vi "5_SPA_KEYSIGHT_rabi_measurements_(SPA_Aver_Mult_traces-Rabi).vi"() -> ()   [LabVIEW 2013]
uses:
  <vilib>/Analysis/baseanly.llb/Mean (DBL).vi
  <vilib>/Analysis/NI_AALBase.lvlib
panel:
  in  "Connection":T1={"Type"=0, "VISA"="TCPIP0::192.168.0.8::inst0::INSTR", "GPIB"="10"} {"Type" items=["VISA", "GPIB"]}
  out "x/y":dbl
  out "Normalised":dbl[][](graph)
  out "(Current)":i32=103
  in  "Program to run":u16(ring) items=["Rabi", "T2"]
  in  "?":enum32{"VNA", "SPA"}(tab)
  in  "Center Freq (Hz)":dbl=6953330000.0 caption="Center Freq (Hz):" format="%#.6p"
  in  "VNA Power dBm":dbl=-10.0 caption="VNA Power (dBm)" format="%#.3f"
  in  "Points":i32=2147483647 caption="Center Freq (Hz):"
  in  "Span (Hz)":dbl=6953330000.0 caption="Center Freq (Hz):" format="%#.6p"
  in  "RBW (Hz)":dbl=6953330000.0 caption="Center Freq (Hz):" format="%#.6p"
  in  "VBW (Hz)":dbl=6953330000.0 caption="Center Freq (Hz):" format="%#.6p"
  in  "Averages":u32=251
  out "Background":dbl[][](graph)
  out "Signal":dbl[][](graph)
  out "(Current)":i32=103
  out "Background":dbl[](graph)
  in  "Numeric":u32=251
  in  "Start (ns)":dbl=2.0
  in  "End (ns)":dbl=52.0
  out "Normalised Signal":dbl[][](graph)
  out "Signal":dbl[](graph)
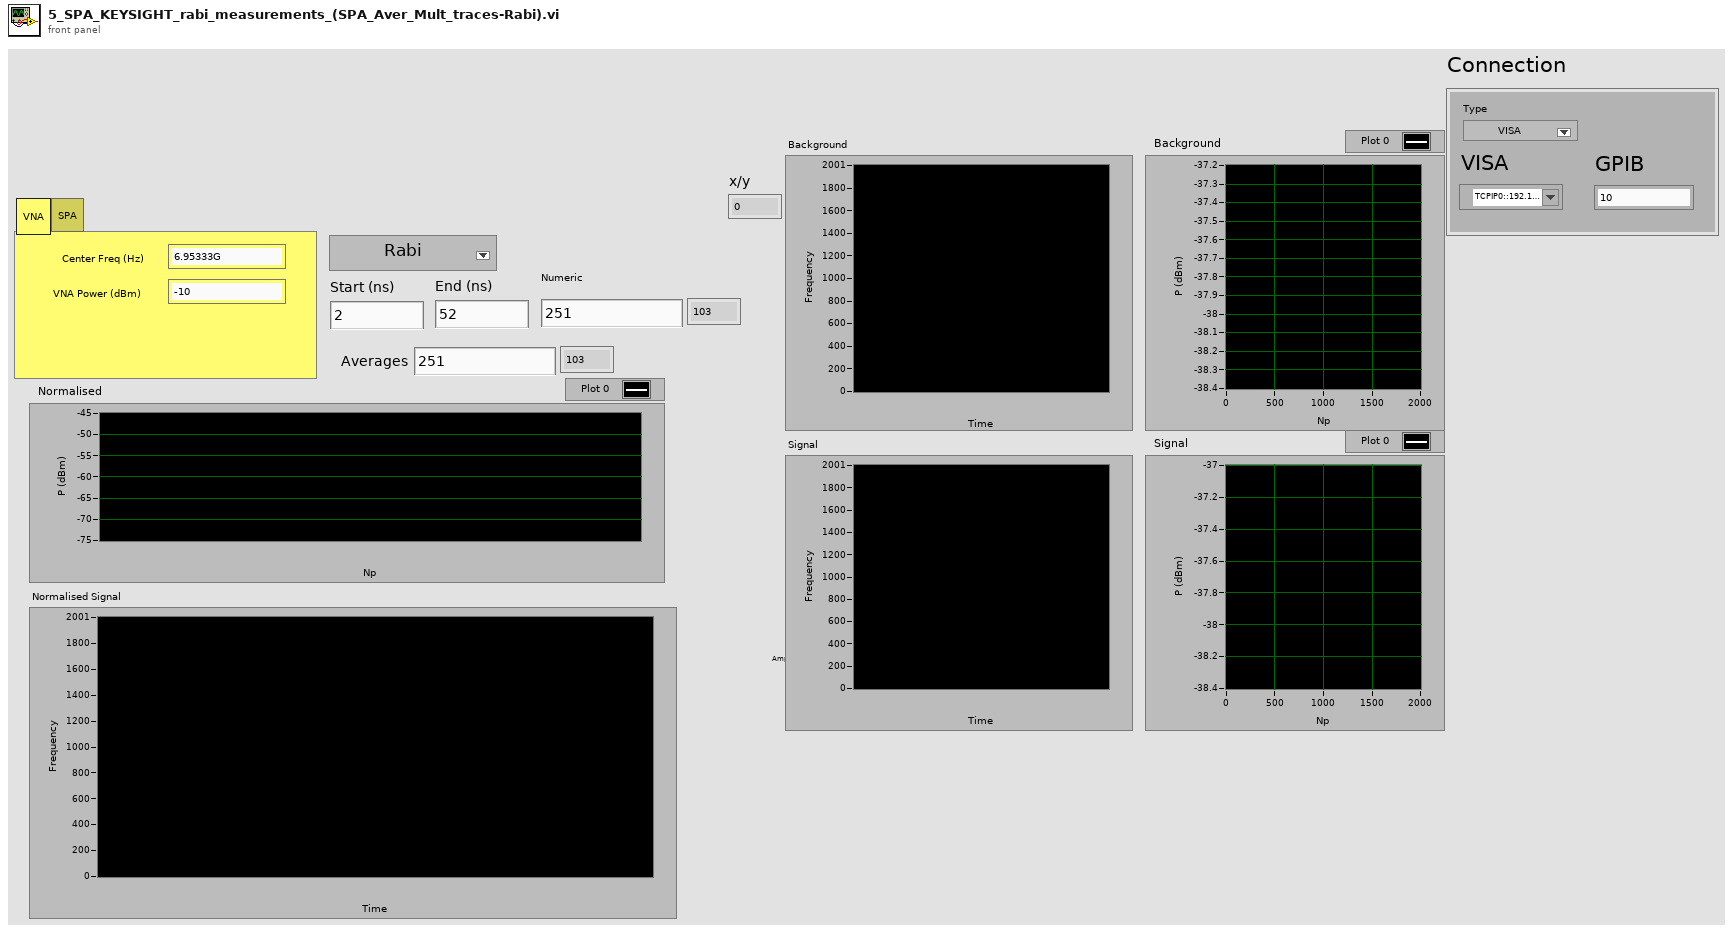
[diagram p1: front panel]
types:
  T1 = cluster{"Type":u16, "VISA":refnum<visa-resource-name>, "GPIB":string}
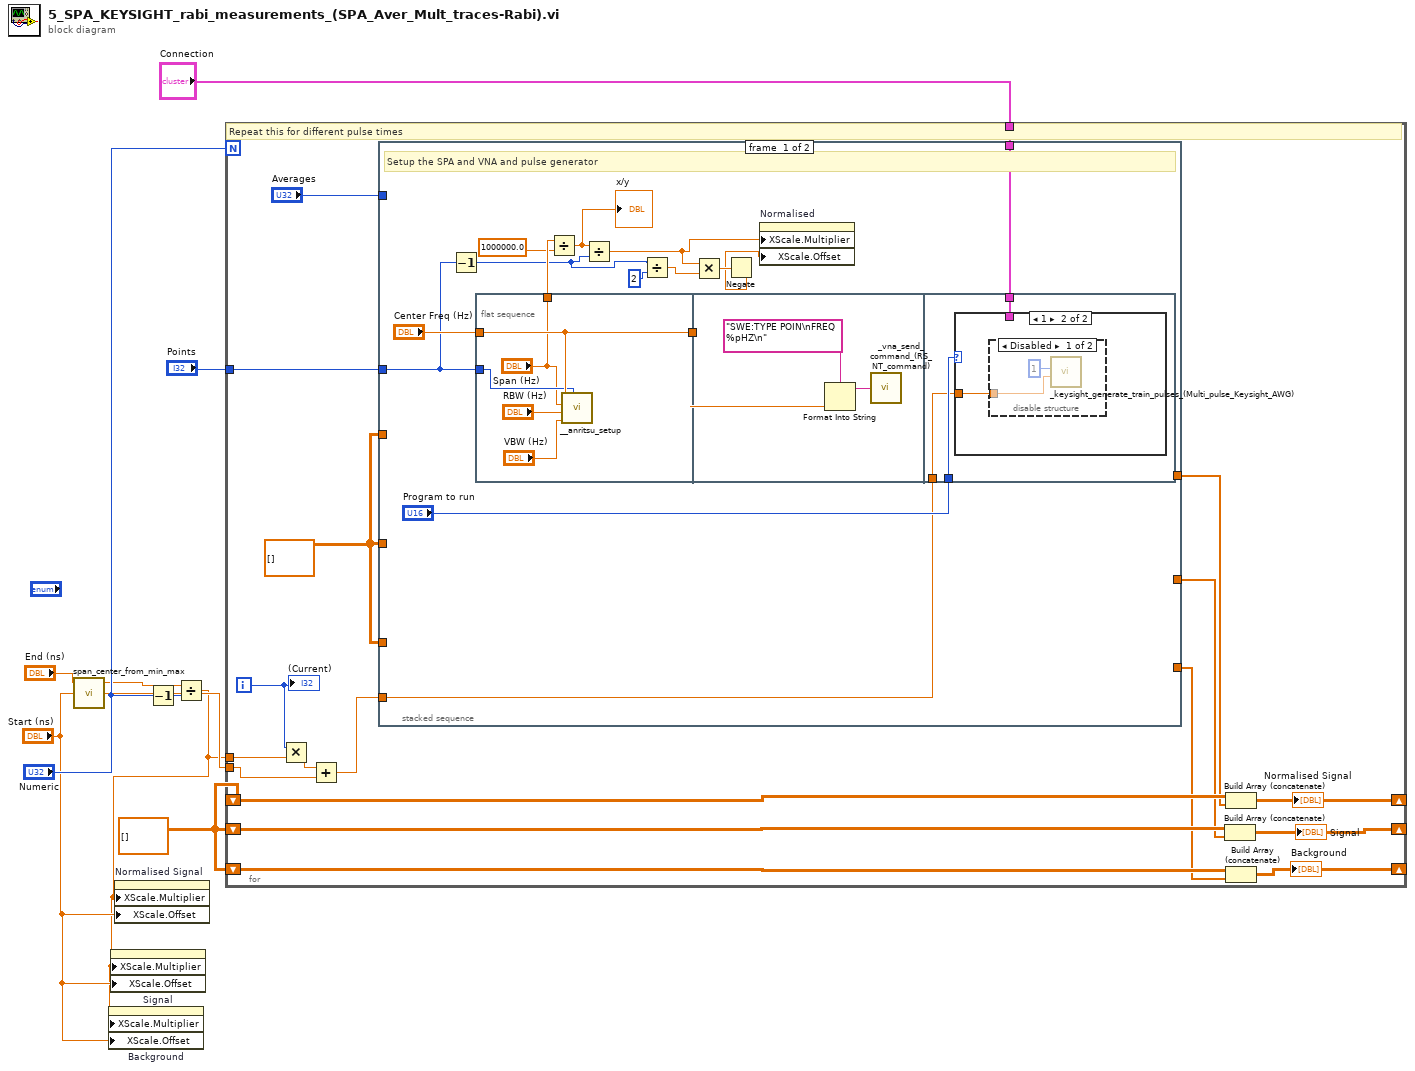
[diagram p0: block diagram]
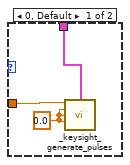
[diagram p2: hidden frame]
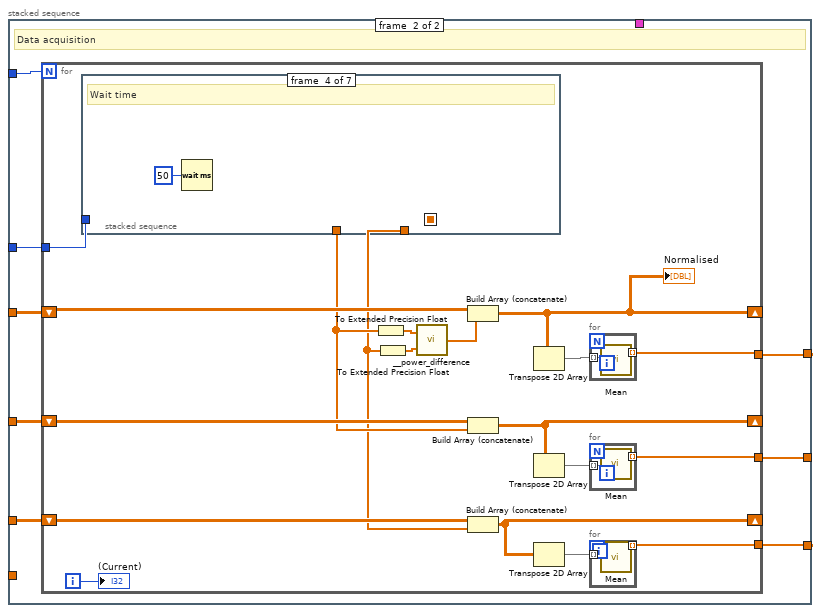
[diagram p4: hidden frame]
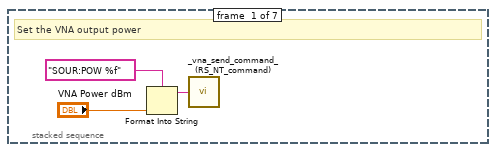
[diagram p5: hidden frame]
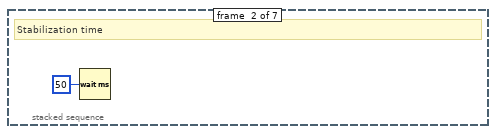
[diagram p6: hidden frame]
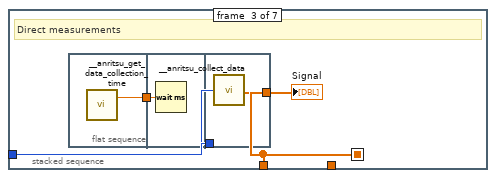
[diagram p7: hidden frame]
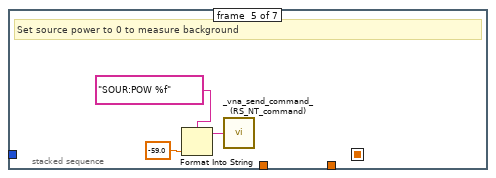
[diagram p8: hidden frame]
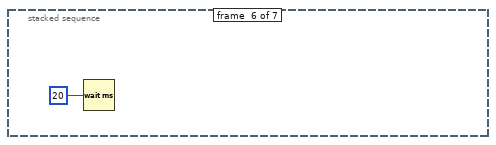
[diagram p9: hidden frame]
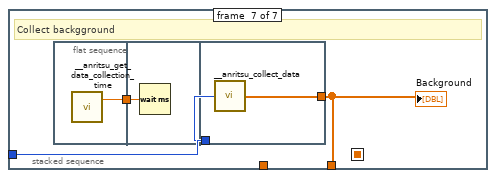
[diagram p10: hidden frame]
diagram:
  w5 = dbl[][] [] ("initialized array")
  n1 = call "span_center_from_min_max.vi"("Begin"="Start (ns)", "End"="End (ns)") -> ("Difference (abs)"=w6:dbl)  [unwired: 1 in, 2 out]
  n2 = Decrement(x="Numeric") -> (x-1=w9:u32)
  n3 = Divide(x=w6, y=w9) -> (x/y=w2:dbl)
  n4 = property on="Background" class="IntGraph (strict)"("XScale.Multiplier"=w2, "XScale.Offset"="Start (ns)") -> ()  [unwired: 2 in, 2 out]
  n5 = property on="Signal" class="IntGraph (strict)"("XScale.Multiplier"=w2, "XScale.Offset"="Start (ns)") -> ()  [unwired: 2 in, 2 out]
  n6 = property on="Normalised Signal" class="IntGraph (strict)"("XScale.Multiplier"=w2, "XScale.Offset"="Start (ns)") -> ()  [unwired: 2 in, 2 out]
  n7 = for {
    N: "Numeric" -> [_]
    shift-right: [w24] -> _
    shift-left: w5 -> [w26]
    tunnel: w2 -> [w13]
    tunnel: "Start (ns)" -> [w15]
    shift-right: [w19] -> _
    shift-left: w5 -> [w23]
    shift-right: [w18] -> _
    shift-left: w5 -> [w22]
    tunnel: "Points" -> [w11]
    tunnel: "Connection" -> [w10]
    i -> [w14]
    w17 = dbl[][] [] ("initialized array")
    # "Repeat this for different pulse times"
    n8 = Multiply(x=w14, y=w13) -> (x*y=w12:dbl)
    n9 = Add(x=w12, y=w15) -> (x+y=w16:dbl)
    n10 = stacked-sequence {
      tunnel: "Averages" -> [_ w67]
      tunnel: [_ w66] -> w25
      tunnel: [_ w65] -> w21
      tunnel: [_ w64] -> w20
      tunnel: w17 -> [_ w63]
      tunnel: w17 -> [_ w62]
      tunnel: w17 -> [_ w61]
      tunnel: w16 -> [w40 _]
      tunnel: w11 -> [w30 w60]
      tunnel: w10 -> [w28 _]
      frame #0 {
        # "Setup the SPA and VNA and pulse generator"
        n11 = Decrement(x=w30) -> (x-1=w29:i32)
        n12 = flat-sequence {
          tunnel: w30 -> [w46]
          tunnel: "Center Freq (Hz)" -> [w47]
          tunnel: [w47] -> w42
          tunnel: ["Span (Hz)"] -> w38
          tunnel: w42 -> [w48]
          tunnel: "Program to run" -> [w53]
          tunnel: w40 -> [w52]
          tunnel: w28 -> [w51]
          frame #0 {
            n13 = call "__anritsu_setup.vi"("Center Freq (Hz)"=w47, "Span (Hz)"="Span (Hz)", "RBW (Hz)"="RBW (Hz)", "VBW (Hz)"="VBW (Hz)", "Points"=w46) -> ()  [unwired: 1 out]
          }
          frame #1 {
            n14 = Format Into String(format string="SWE:TYPE POIN\nFREQ %pHZ\n" ("Comand"), w48) -> (resulting string=w50:string)  [unwired: 2 in, 1 out]
            n15 = call "_vna_send_command_(RS_NT_command).vi"("Comand"=w50) -> ()  [unwired: 4 in, 1 out]
          }
          frame #2 {
            n16 = case shown="1" w53 {
              tunnel: w52 -> [w55 w57]
              tunnel: w51 -> [w54 _]
              frame 0, Default {
                w56 = 0.0 ("x")
                n17 = call "_keysight_generate_pulses.vi"("Ch1 pulse_width (ns)"=w55, "Connection"=w54, "Ch2 pulse_width (ns)"=w56, "Ch1 pulse_delay (ns)"=w56, "Ch2 pulse_delay (ns)"=w56) -> ()  [unwired: 9 in, 2 out]
              }
              frame 1 {
                n18 = disable-structure shown="Disabled" {
                  disable-tunnel: w57 -> [w58 _]
                  frame Disabled {
                    n19 = call "_keysight_generate_train_pulses_(Multi_pulse_Keysight_AWG).vi"("start (ns)"=w58, "N"=1) -> ()  [unwired: 10 in]
                  }
                  frame Enabled {
                  }
                }
              }
            }
          }
        }
        n20 = Divide(x=w38, y=1000000.0) -> (x/y=w36:dbl)
        "x/y" <- w36
        n21 = Divide(x=w36, y=w29) -> (x/y=w34:dbl)
        n22 = Divide(x=w29, y=2) -> (x/y=w33:dbl)
        n23 = Multiply(x=w34, y=w33) -> (x*y=w32:dbl)
        n24 = Negate(x=w32) -> (-x=w31:dbl)
        n25 = property on="Normalised" class="WFGraph (strict)"("XScale.Multiplier"=w34, "XScale.Offset"=w31) -> ()  [unwired: 2 in, 2 out]
      }
      frame #1 {
        # "Data acquisition"
        n26 = for {
          N: w67 -> [_]
          shift-right: [w68] -> _
          shift-left: w63 -> [w86]
          tunnel: [w84] -> w66
          shift-right: [w78] -> _
          shift-left: w62 -> [w82]
          shift-right: [w77] -> _
          shift-left: w61 -> [w81]
          tunnel: [w76] -> w65
          tunnel: [w75] -> w64
          tunnel: w60 -> [w74]
          i -> [w83]
          n27 = stacked-sequence {
            seq-local: [_ _ w97 _ _ _ _] -> [_ _ _ _ _ _ _]
            tunnel: [_ _ w97 _ _ _ _] -> w72
            tunnel: [_ _ _ _ _ _ w109] -> w69
            tunnel: w74 -> [_ _ w99 _ _ _ w111]
            frame #0 {
              # "Set the VNA output power"
              n28 = Format Into String(format string="SOUR:POW %f" ("Comand"), "VNA Power dBm") -> (resulting string=w94:string)  [unwired: 2 in, 1 out]
              n29 = call "_vna_send_command_(RS_NT_command).vi"("Comand"=w94) -> ()  [unwired: 4 in, 1 out]
            }
            frame #1 {
              # "Stabilization time"
              n30 = Wait (ms)(milliseconds to wait=u32 50) -> ()  [unwired: 1 out]
            }
            frame #2 {
              # "Direct measurements"
              n31 = flat-sequence {
                tunnel: [w100] -> w98
                tunnel: w98 -> [w101]
                tunnel: [w103] -> w97
                tunnel: w99 -> [w102]
                frame #0 {
                  n32 = call "__anritsu_get_data_collection_time.vi"() -> ("Time to wait (ms)"=w100:dbl)  [unwired: 1 out]
                }
                frame #1 {
                  n33 = Wait (ms)(milliseconds to wait=w101) -> ()  [unwired: 1 out]
                }
                frame #2 {
                  n34 = call "__anritsu_collect_data.vi"("Points to read"=w102) -> ("Data out"=w103:dbl[])
                }
              }
              "Signal" <- w97
            }
            frame #3 {
              # "Wait time"
              n35 = Wait (ms)(milliseconds to wait=u32 50) -> ()  [unwired: 1 out]
            }
            frame #4 {
              # "Set source power to 0 to measure background"
              n36 = Format Into String(format string="SOUR:POW %f" ("Comand"), -59.0 ("input 2")) -> (resulting string=w106:string)  [unwired: 2 in, 1 out]
              n37 = call "_vna_send_command_(RS_NT_command).vi"("Comand"=w106) -> ()  [unwired: 4 in, 1 out]
            }
            frame #5 {
              n38 = Wait (ms)(milliseconds to wait=u32 20) -> ()  [unwired: 1 out]
            }
            frame #6 {
              # "Collect backgground"
              n39 = flat-sequence {
                tunnel: [w112] -> w110
                tunnel: w110 -> [w113]
                tunnel: w111 -> [w115]
                tunnel: [w114] -> w109
                frame #0 {
                  n40 = call "__anritsu_get_data_collection_time.vi"() -> ("Time to wait (ms)"=w112:dbl)  [unwired: 1 out]
                }
                frame #1 {
                  n41 = Wait (ms)(milliseconds to wait=w113) -> ()  [unwired: 1 out]
                }
                frame #2 {
                  n42 = call "__anritsu_collect_data.vi"("Points to read"=w115) -> ("Data out"=w114:dbl[])
                }
              }
              "Background" <- w109
            }
          }
          n43 = To Extended Precision Float(1:w72) -> (0:w71:ext[])
          n44 = To Extended Precision Float(1:w69) -> (0:w70:ext[])
          n45 = call "__power_difference.vi"("Power Low dBm"=w70, "Power High dBm"=w71) -> ("Power Difference dBm"=w73:dbl[])
          n46 = Build Array (concatenate)(w86, w73) -> (w68:dbl[][])
          "Normalised" <- w68
          n47 = Build Array (concatenate)(w82, w72) -> (w78:dbl[][])
          n48 = Build Array (concatenate)(w81, w69) -> (w77:dbl[][])
          n49 = Transpose 2D Array(2D array=w68) -> (transposed array=w85:dbl[][])
          n50 = Transpose 2D Array(2D array=w78) -> (transposed array=w80:dbl[][])
          n51 = Transpose 2D Array(2D array=w77) -> (transposed array=w79:dbl[][])
          n52 = for {
            tunnel: w85 -> [w92] mode=indexing
            tunnel: [w91] -> w84 mode=indexing
            n53 = call-poly <vilib>:"Mean.vi"("X"=w92) -> ("mean"=w91:dbl)  [unwired: 1 out]
          }
          n54 = for {
            tunnel: w80 -> [w90] mode=indexing
            tunnel: [w89] -> w76 mode=indexing
            n55 = call-poly <vilib>:"Mean.vi"("X"=w90) -> ("mean"=w89:dbl)  [unwired: 1 out]
          }
          n56 = for {
            tunnel: w79 -> [w88] mode=indexing
            tunnel: [w87] -> w75 mode=indexing
            n57 = call-poly <vilib>:"Mean.vi"("X"=w88) -> ("mean"=w87:dbl)  [unwired: 1 out]
          }
          "(Current)" <- w83
        }
      }
    }
    n58 = Build Array (concatenate)(w23, w21) -> (w19:dbl[][])
    "Signal" <- w19
    n59 = Build Array (concatenate)(w26, w25) -> (w24:dbl[][])
    "Normalised Signal" <- w24
    n60 = Build Array (concatenate)(w22, w20) -> (w18:dbl[][])
    "Background" <- w18
    "(Current)" <- w14
  }
